vi "OFDM_SuperpositionedBitDetect - Diff Mod.vi"(0 "Input symbols":cdb[](array[numeric]) format="%.2f", 1 "Modulation type":T1(ring), 2 "Modulation type 2":T1(ring), 3 "error in (no error)":errorcluster, 4 "SIC Amp":dbl(slide)=1.0 scale=1.0..5.0) -> (5 "Base Bits":i8[](array[numeric]), 6 "SC Symbols":cdb[](array[numeric]), 7 "SC Bits":i8[](array[numeric]), 10 "error out":errorcluster)   [LabVIEW 2022 SP3]
uses:
  <vilib>/addons/Modulation/Digital/General/MT Map QAM Symbols to Bits.vi
  <vilib>/addons/Modulation/Digital/General/MT Map Bits to QAM Symbols.vi
  <vilib>/addons/Modulation/Digital/General/MT Map PSK Symbols to Bits.vi
  <vilib>/addons/Modulation/Digital/General/MT Map Bits to PSK Symbols.vi
  <vilib>/addons/Modulation/niDMT.lvlib
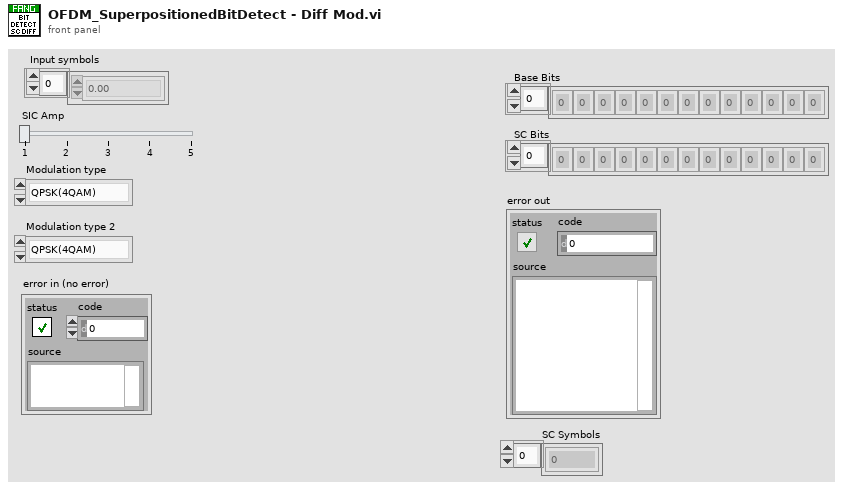
[diagram p1: front panel]
types:
  T1 = enum16{"QPSK(4QAM)", "64QAM", "16QAM", "BPSK", "BPSK Vertical"}
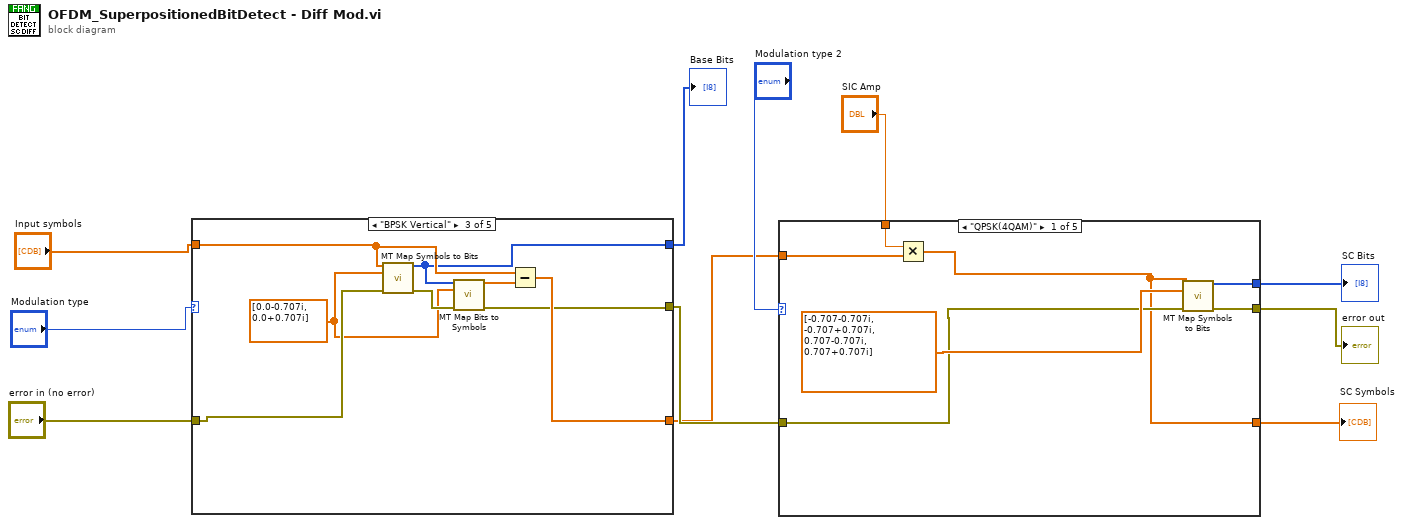
[diagram p0: block diagram]
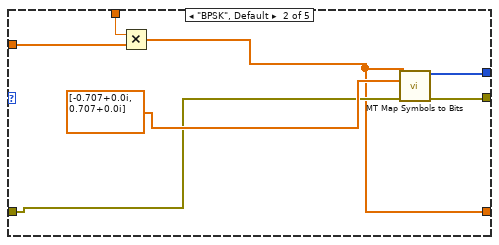
[diagram p2: hidden frame]
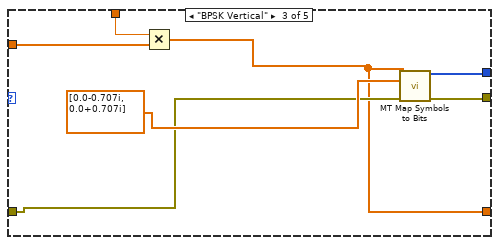
[diagram p3: hidden frame]
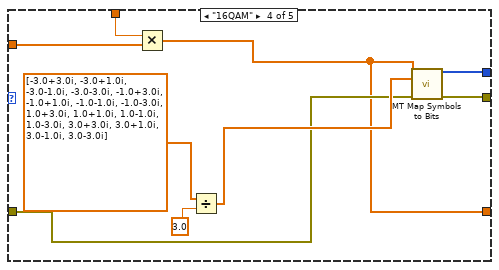
[diagram p4: hidden frame]
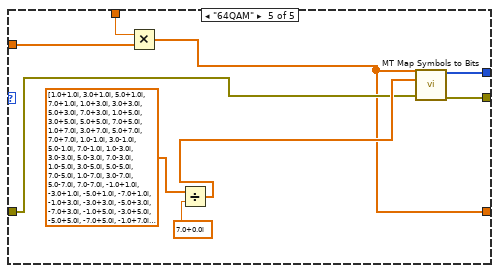
[diagram p5: hidden frame]
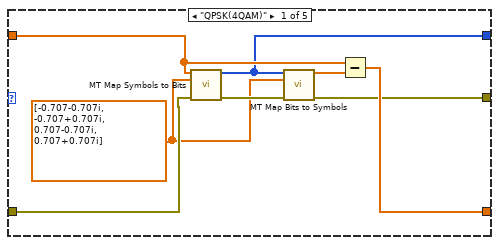
[diagram p6: hidden frame]
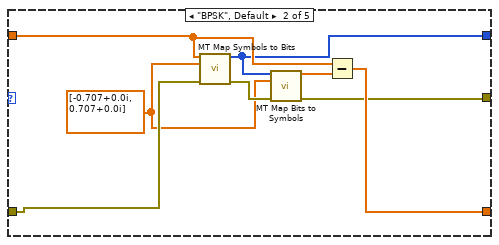
[diagram p7: hidden frame]
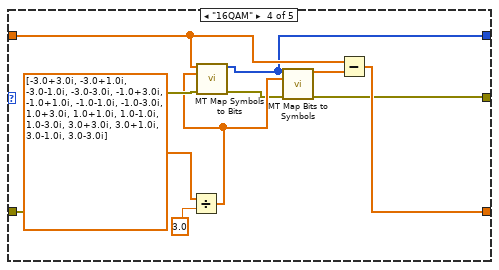
[diagram p8: hidden frame]
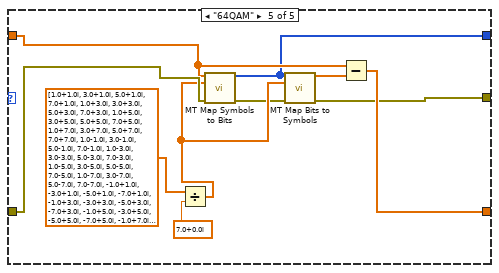
[diagram p9: hidden frame]
diagram:
  n1 = case shown="\"BPSK Vertical\"" "Modulation type" {
    tunnel: "Input symbols" -> [w16 w23 w31 w40 w50]
    tunnel: "error in (no error)" -> [w19 w27 w35 w45 w53]
    tunnel: [w12 w20 w28 w36 w46] -> w4
    tunnel: [w14 w22 w30 w38 w48] -> w8
    tunnel: [w13 w21 w29 w37 w47] -> w3
    frame "QPSK(4QAM)" {
      w15 = cdb[] [-0.707-0.707i, -0.707+0.707i, 0.707-0.707i, 0.707+0.707i] ("symbol map")
      n2 = call-poly <vilib>:"MT Map Symbols to Bits.vi"("symbols"=w16, "symbol map"=w15, "error in (no error)"=w19) -> ("output bit stream"=w14:i8[], "error out"=w18:errorcluster)  [unwired: 11 in]
      n3 = call-poly <vilib>:"MT Map Bits to Symbols.vi"("input bit stream"=w14, "symbol map"=w15, "error in (no error)"=w18) -> ("symbols"=w17:cdb[], "error out"=w12:errorcluster)  [unwired: 11 in]
      n4 = Subtract(x=w16, y=w17) -> (x-y=w13:cdb[])
    }
    frame "BPSK", Default {
      w25 = cdb[] [-0.707+0.0i, 0.707+0.0i] ("symbol map")
      n5 = call-poly <vilib>:"MT Map Symbols to Bits.vi"("symbols"=w23, "symbol map"=w25, "error in (no error)"=w27) -> ("output bit stream"=w22:i8[], "error out"=w26:errorcluster)  [unwired: 11 in]
      n6 = call-poly <vilib>:"MT Map Bits to Symbols.vi"("input bit stream"=w22, "symbol map"=w25, "error in (no error)"=w26) -> ("symbols"=w24:cdb[], "error out"=w20:errorcluster)  [unwired: 11 in]
      n7 = Subtract(x=w23, y=w24) -> (x-y=w21:cdb[])
    }
    frame "BPSK Vertical" {
      w33 = cdb[] [0.0-0.707i, 0.0+0.707i] ("symbol map")
      n8 = call-poly <vilib>:"MT Map Symbols to Bits.vi"("symbols"=w31, "symbol map"=w33, "error in (no error)"=w35) -> ("output bit stream"=w30:i8[], "error out"=w34:errorcluster)  [unwired: 11 in]
      n9 = call-poly <vilib>:"MT Map Bits to Symbols.vi"("input bit stream"=w30, "symbol map"=w33, "error in (no error)"=w34) -> ("symbols"=w32:cdb[], "error out"=w28:errorcluster)  [unwired: 11 in]
      n10 = Subtract(x=w31, y=w32) -> (x-y=w29:cdb[])
    }
    frame "16QAM" {
      n11 = Divide(x=cdb[] [-3.0+3.0i, -3.0+1.0i, -3.0-1.0i, -3.0-3.0i, -1.0+3.0i, -1.0+1.0i, -1.0-1.0i, -1.0-3.0i, 1.0+3.0i, 1.0+1.0i, 1.0-1.0i, 1.0-3.0i, 3.0+3.0i, 3.0+1.0i, 3.0-1.0i, 3.0-3.0i] ("symbol map"), y=3.0) -> (x/y=w42:cdb[])
      n12 = call-poly <vilib>:"MT Map Symbols to Bits.vi"("symbols"=w40, "symbol map"=w42, "error in (no error)"=w45) -> ("output bit stream"=w38:i8[], "error out"=w39:errorcluster)  [unwired: 11 in]
      n13 = call-poly <vilib>:"MT Map Bits to Symbols.vi"("input bit stream"=w38, "symbol map"=w42, "error in (no error)"=w39) -> ("symbols"=w41:cdb[], "error out"=w36:errorcluster)  [unwired: 11 in]
      n14 = Subtract(x=w40, y=w41) -> (x-y=w37:cdb[])
    }
    frame "64QAM" {
      n15 = Divide(x=cdb[] [1.0+1.0i, 3.0+1.0i, 5.0+1.0i, 7.0+1.0i, 1.0+3.0i, 3.0+3.0i, 5.0+3.0i, 7.0+3.0i, 1.0+5.0i, 3.0+5.0i, 5.0+5.0i, 7.0+5.0i, 1.0+7.0i, 3.0+7.0i, 5.0+7.0i, 7.0+7.0i, 1.0-1.0i, 3.0-1.0i, 5.0-1.0i, 7.0-1.0i, 1.0-3.0i, 3.0-3.0i, 5.0-3.0i, 7.0-3.0i, 1.0-5.0i, 3.0-5.0i, 5.0-5.0i, 7.0-5.0i, 1.0-7.0i, 3.0-7.0i, 5.0-7.0i, 7.0-7.0i, -1.0+1.0i, -3.0+1.0i, -5.0+1.0i, -7.0+1.0i, -1.0+3.0i, -3.0+3.0i, -5.0+3.0i, -7.0+3.0i, -1.0+5.0i, -3.0+5.0i, -5.0+5.0i, -7.0+5.0i, -1.0+7.0i, -3.0+7.0i, -5.0+7.0i, -7.0+7.0i, -1.0-1.0i, -3.0-1.0i, -5.0-1.0i, -7.0-1.0i, -1.0-3.0i, -3.0-3.0i, -5.0-3.0i, -7.0-3.0i, -1.0-5.0i, -3.0-5.0i, -5.0-5.0i, -7.0-5.0i, -1.0-7.0i, -3.0-7.0i, -5.0-7.0i, -7.0-7.0i] ("appended array"), y=cdb 7.0+0.0i) -> (x/y=w52:cdb[])
      n16 = call-poly <vilib>:"MT Map Symbols to Bits.vi"("symbols"=w50, "symbol map"=w52, "error in (no error)"=w53) -> ("output bit stream"=w48:i8[], "error out"=w49:errorcluster)  [unwired: 11 in]
      n17 = call-poly <vilib>:"MT Map Bits to Symbols.vi"("input bit stream"=w48, "symbol map"=w52, "error in (no error)"=w49) -> ("symbols"=w51:cdb[], "error out"=w46:errorcluster)  [unwired: 11 in]
      n18 = Subtract(x=w50, y=w51) -> (x-y=w47:cdb[])
    }
  }
  "Base Bits" <- w8
  n19 = case shown="\"QPSK(4QAM)\"" "Modulation type 2" {
    tunnel: w3 -> [w58 w65 w70 w78 w88]
    tunnel: w4 -> [w59 w66 w73 w80 w89]
    tunnel: [w60 w68 w75 w83 w91] -> w2
    tunnel: [w62 w69 w76 w82 w90] -> w6
    tunnel: [w56 w64 w72 w79 w87] -> w5
    tunnel: "SIC Amp" -> [w57 w63 w71 w77 w86]
    frame "QPSK(4QAM)" {
      n20 = Multiply(x=w57, y=w58) -> (x*y=w56:cdb[])
      n21 = call-poly <vilib>:"MT Map Symbols to Bits.vi"("symbols"=w56, "symbol map"=cdb[] [-0.707-0.707i, -0.707+0.707i, 0.707-0.707i, 0.707+0.707i], "error in (no error)"=w59) -> ("output bit stream"=w60:i8[], "error out"=w62:errorcluster)  [unwired: 11 in]
    }
    frame "BPSK", Default {
      n22 = Multiply(x=w63, y=w65) -> (x*y=w64:cdb[])
      n23 = call-poly <vilib>:"MT Map Symbols to Bits.vi"("symbols"=w64, "symbol map"=cdb[] [-0.707+0.0i, 0.707+0.0i], "error in (no error)"=w66) -> ("output bit stream"=w68:i8[], "error out"=w69:errorcluster)  [unwired: 11 in]
    }
    frame "BPSK Vertical" {
      n24 = Multiply(x=w71, y=w70) -> (x*y=w72:cdb[])
      n25 = call-poly <vilib>:"MT Map Symbols to Bits.vi"("symbols"=w72, "symbol map"=cdb[] [0.0-0.707i, 0.0+0.707i], "error in (no error)"=w73) -> ("output bit stream"=w75:i8[], "error out"=w76:errorcluster)  [unwired: 11 in]
    }
    frame "16QAM" {
      n26 = Multiply(x=w77, y=w78) -> (x*y=w79:cdb[])
      n27 = Divide(x=cdb[] [-3.0+3.0i, -3.0+1.0i, -3.0-1.0i, -3.0-3.0i, -1.0+3.0i, -1.0+1.0i, -1.0-1.0i, -1.0-3.0i, 1.0+3.0i, 1.0+1.0i, 1.0-1.0i, 1.0-3.0i, 3.0+3.0i, 3.0+1.0i, 3.0-1.0i, 3.0-3.0i] ("symbol map"), y=3.0) -> (x/y=w81:cdb[])
      n28 = call-poly <vilib>:"MT Map Symbols to Bits.vi"("symbols"=w79, "symbol map"=w81, "error in (no error)"=w80) -> ("output bit stream"=w83:i8[], "error out"=w82:errorcluster)  [unwired: 11 in]
    }
    frame "64QAM" {
      n29 = Multiply(x=w86, y=w88) -> (x*y=w87:cdb[])
      n30 = Divide(x=cdb[] [1.0+1.0i, 3.0+1.0i, 5.0+1.0i, 7.0+1.0i, 1.0+3.0i, 3.0+3.0i, 5.0+3.0i, 7.0+3.0i, 1.0+5.0i, 3.0+5.0i, 5.0+5.0i, 7.0+5.0i, 1.0+7.0i, 3.0+7.0i, 5.0+7.0i, 7.0+7.0i, 1.0-1.0i, 3.0-1.0i, 5.0-1.0i, 7.0-1.0i, 1.0-3.0i, 3.0-3.0i, 5.0-3.0i, 7.0-3.0i, 1.0-5.0i, 3.0-5.0i, 5.0-5.0i, 7.0-5.0i, 1.0-7.0i, 3.0-7.0i, 5.0-7.0i, 7.0-7.0i, -1.0+1.0i, -3.0+1.0i, -5.0+1.0i, -7.0+1.0i, -1.0+3.0i, -3.0+3.0i, -5.0+3.0i, -7.0+3.0i, -1.0+5.0i, -3.0+5.0i, -5.0+5.0i, -7.0+5.0i, -1.0+7.0i, -3.0+7.0i, -5.0+7.0i, -7.0+7.0i, -1.0-1.0i, -3.0-1.0i, -5.0-1.0i, -7.0-1.0i, -1.0-3.0i, -3.0-3.0i, -5.0-3.0i, -7.0-3.0i, -1.0-5.0i, -3.0-5.0i, -5.0-5.0i, -7.0-5.0i, -1.0-7.0i, -3.0-7.0i, -5.0-7.0i, -7.0-7.0i] ("appended array"), y=cdb 7.0+0.0i) -> (x/y=w92:cdb[])
      n31 = call-poly <vilib>:"MT Map Symbols to Bits.vi"("symbols"=w87, "symbol map"=w92, "error in (no error)"=w89) -> ("output bit stream"=w91:i8[], "error out"=w90:errorcluster)  [unwired: 11 in]
    }
  }
  "SC Bits" <- w2
  "error out" <- w6
  "SC Symbols" <- w5
